vi "Personality_Reader.vi"(0 "GEA2 Reference In":refnum<k24>, 1 "GEA Inputs":T1 {"Destination" format="%.0x"; "Source" format="%.0x"}, 2 "Standalone?":bool, 11 "Error In":errorcluster) -> (4 "GEA2 Reference Out":refnum<k24>, 6 "Personality":string, 15 "Error Out":errorcluster)   [LabVIEW 2016, in "TLMB.lvlib"]
doc: "This vi can be used to read ERD every 1 sec for user selected repeat counts."
uses:
  Projects/TLMB.lvlib
  Q:/Common/DLLs/GEA3/GeaCommunication.dll
  Common/DLLs/GEA3/GeaCommunication.dll
  Common/LabVIEW GEA2 Toolkit/LabVIEW_GEA2_Toolkit.lvlibp/type defs/Source_Destination.ctl
  Common/LabVIEW GEA2 Toolkit/LabVIEW_GEA2_Toolkit.lvlibp/type defs/ERD Read Data In.ctl
  Common/LabVIEW GEA2 Toolkit/LabVIEW_GEA2_Toolkit.lvlibp/type defs/Data Type.ctl
  Common/LabVIEW GEA2 Toolkit/LabVIEW_GEA2_Toolkit.lvlibp
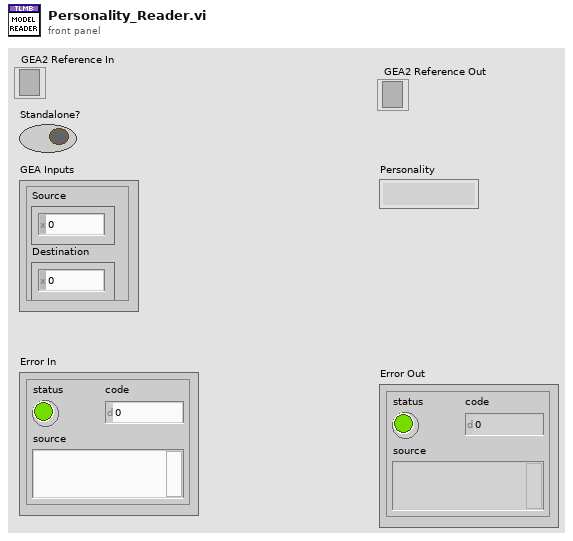
[diagram p1: front panel]
types:
  T1 = typedef "LabVIEW_GEA2_Toolkit.lvlibp/Source_Destination.ctl" = cluster{"Source":u8, "Destination":u8}
  T2 = typedef "LabVIEW_GEA2_Toolkit.lvlibp/ERD Read Data In.ctl" = cluster{"ERD Number":u16, "Data Type":T3}
  T3 = typedef "LabVIEW_GEA2_Toolkit.lvlibp/Data Type.ctl" = enum16{"string", "boolean", "uint8_t", "uint16_t", "uint32_t", "uint64_t", "int8_t", "int16_t", "int32_t", "int64_t"}
  T4 = typedef "LabVIEW_GEA2_Toolkit.lvlibp/ERD Read Data Out.ctl" = cluster{"ERD Number":u16, "Data":string}
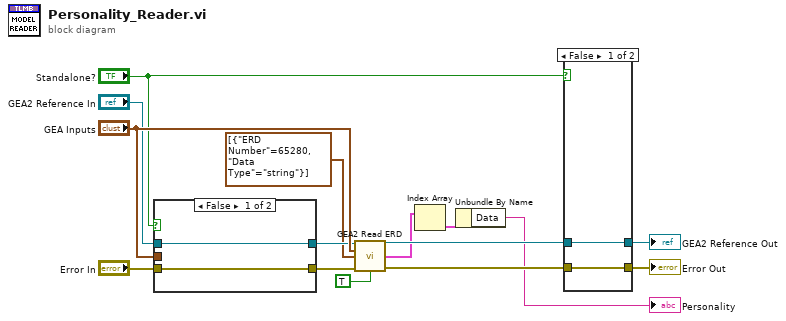
[diagram p0: block diagram]
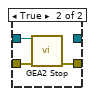
[diagram p2: hidden frame]
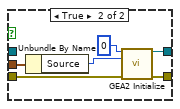
[diagram p3: hidden frame]
diagram:
  n1 = case shown="False" "Standalone?" {
    tunnel: "Error In" -> [w16 w23]
    tunnel: [w16 w22] -> w10
    tunnel: "GEA2 Reference In" -> [w17 _]
    tunnel: [w17 w21] -> w9
    tunnel: "GEA Inputs" -> [_ w19]
    frame False {
    }
    frame True {
      n2 = Unbundle By Name(w19) -> ("Source"=w20:u8)
      n3 = call "GEA2 Initialize.vi"("Board Index"=0, "Source Address"=w20, "error in"=w23) -> ("GEA2 Reference Out"=w21:refnum<k24>, "error out"=w22:errorcluster)  [unwired: 10 in, 1 out]
    }
  }
  n4 = call "GEA2 Read ERD.vi"("GEA2 Reference In"=w9, "GEA Inputs"="GEA Inputs", "Read ERD List"=T2[] [{"ERD Number"=65280, "Data Type"=enum."string"}], "Error In"=w10, "Verify ERD Response?"=TRUE) -> ("GEA2 Reference Out"=w6:refnum<k24>, "ERD Data Out"=w4:T4[], "Error Out"=w7:errorcluster)  [unwired: 7 in, 1 out]
  n5 = Index Array(array=w4) -> (element=w3:T4)  [unwired: 1 in]
  n6 = Unbundle By Name(w3) -> ("Data"=→"Personality":string)
  n7 = case shown="False" "Standalone?" {
    tunnel: w7 -> [w24 w27]
    tunnel: [w24 w26] -> w14
    tunnel: w6 -> [w25 w28]
    tunnel: [w25 _] -> w8
    frame False {
    }
    frame True {
      n8 = call "GEA2 Stop.vi"("GEA2 Reference In"=w28, "Error In"=w27) -> ("Error Out"=w26:errorcluster)  [unwired: 13 in]
    }
  }
  "Error Out" <- w14
  "GEA2 Reference Out" <- w8
